vi "Niveau.vi"(8 "error in (no error)":errorcluster, 10 "AngleTable":dbl[](array[numeric]), 11 "Axis entrant":dbl[][](array[numeric])) -> (0 "error out":errorcluster, 3 "Axis sortant":dbl[][](array[numeric]))   [LabVIEW 2019]
uses:
  <vilib>/myRIO/Instrument Drivers/Onboard IO/DIO/typedefs/DIO Reference.ctl
  <vilib>/myRIO/Common/Instrument Driver Framework/Utilities/typedefs/myRIO Generic Hardware Reference.ctl
  <vilib>/myRIO/Common/Instrument Driver Framework/Utilities/typedefs/Hardware Version Enum.ctl
  <vilib>/myRIO/Common/Instrument Driver Framework/Utilities/typedefs/myRIO v1.0 Reference.ctl
  <vilib>/myRIO/Common/Instrument Driver Framework/Utilities/typedefs/Generic FPGA Reference.ctl
  <vilib>/myRIO/Common/Instrument Driver Framework/myRIO v1.0/DIO/typedefs/DIO Channels List.ctl
  <vilib>/myRIO/Common/Instrument Driver Framework/myRIO v1.0/DIO/typedefs/DIO Channels Enum.ctl
  <vilib>/userDefined/High Color/nirio_resource_hc.ctl
  <vilib>/myRIO/Common/Instrument Driver Framework/Utilities/vis/Is FPGA Ref Available.vi
  <vilib>/myRIO/Common/Instrument Driver Framework/myRIO v1.0/DIO/vis/myRIO v1.1 Open DIO.vi
  <vilib>/myRIO/Instrument Drivers/Onboard IO/DIO/vis/Write.vi
  <vilib>/myRIO/Common/Instrument Driver Framework/Utilities/vis/Validate Channels.vi
  <vilib>/myRIO/Common/Instrument Driver Framework/myRIO v1.0/DIO/vis/myRIO v1.0 Reserve DIO.vi
  <vilib>/myRIO/Common/Instrument Driver Framework/myRIO v1.0/Resource Manager/vis/myRIO v1.0 Reserve Channel List.vi
  <vilib>/myRIO/Common/Instrument Driver Framework/myRIO v1.0/DIO/vis/myRIO v1.0 Build MUX Configuration DIO.vi
  <vilib>/myRIO/Common/Instrument Driver Framework/myRIO v1.0/Resource Manager/vis/myRIO v1.0 Reserve Channel.vi
  <vilib>/myRIO/Common/Instrument Driver Framework/myRIO v1.0/Resource Manager/vis/myRIO v1.0 Unreserve Channel.vi
  <vilib>/myRIO/Common/Instrument Driver Framework/myRIO v1.0/Resource Manager/vis/myRIO v1.0 Create Configuration List.vi
  <vilib>/myRIO/Common/Instrument Driver Framework/myRIO v1.0/Resource Manager/vis/myRIO v1.0 Build Mutex Name.vi
  <vilib>/Utility/VariantDataType/GetNumericInfo.vi
  <vilib>/Utility/error.llb/Error Cluster From Error Code.vi
  <vilib>/myRIO/Common/Instrument Driver Framework/myRIO v1.0/myRIO v1.1 Open.vi
  <vilib>/myRIO/Common/Instrument Driver Framework/Utilities/vis/IO Manager.vi
  <vilib>/myRIO/Common/Instrument Driver Framework/Utilities/vis/Configuration Manager.vi
  <vilib>/myRIO/Common/Instrument Driver Framework/myRIO v1.0/Resource Manager/vis/myRIO v1.0 Configure IO.vi
  <vilib>/myRIO/Common/Instrument Driver Framework/myRIO v1.0/myRIO v1.0 Close.vi
  <vilib>/myRIO/Common/Instrument Driver Framework/myRIO v1.0/DIO/vis/myRIO v1.0 Write DIO.vi
  <vilib>/myRIO/Express VI/Onboard Devices/LED/LED Express VI.xnode
  <vilib>/myRIO/Instrument Drivers/Onboard IO/DIO/vis/myRIO DIO Open.xnode
  <vilib>/myRIO/Instrument Drivers/Onboard IO/DIO/DIO.lvlib
panel:
  out "DefAngle":dbl
  out "++Angle":dbl
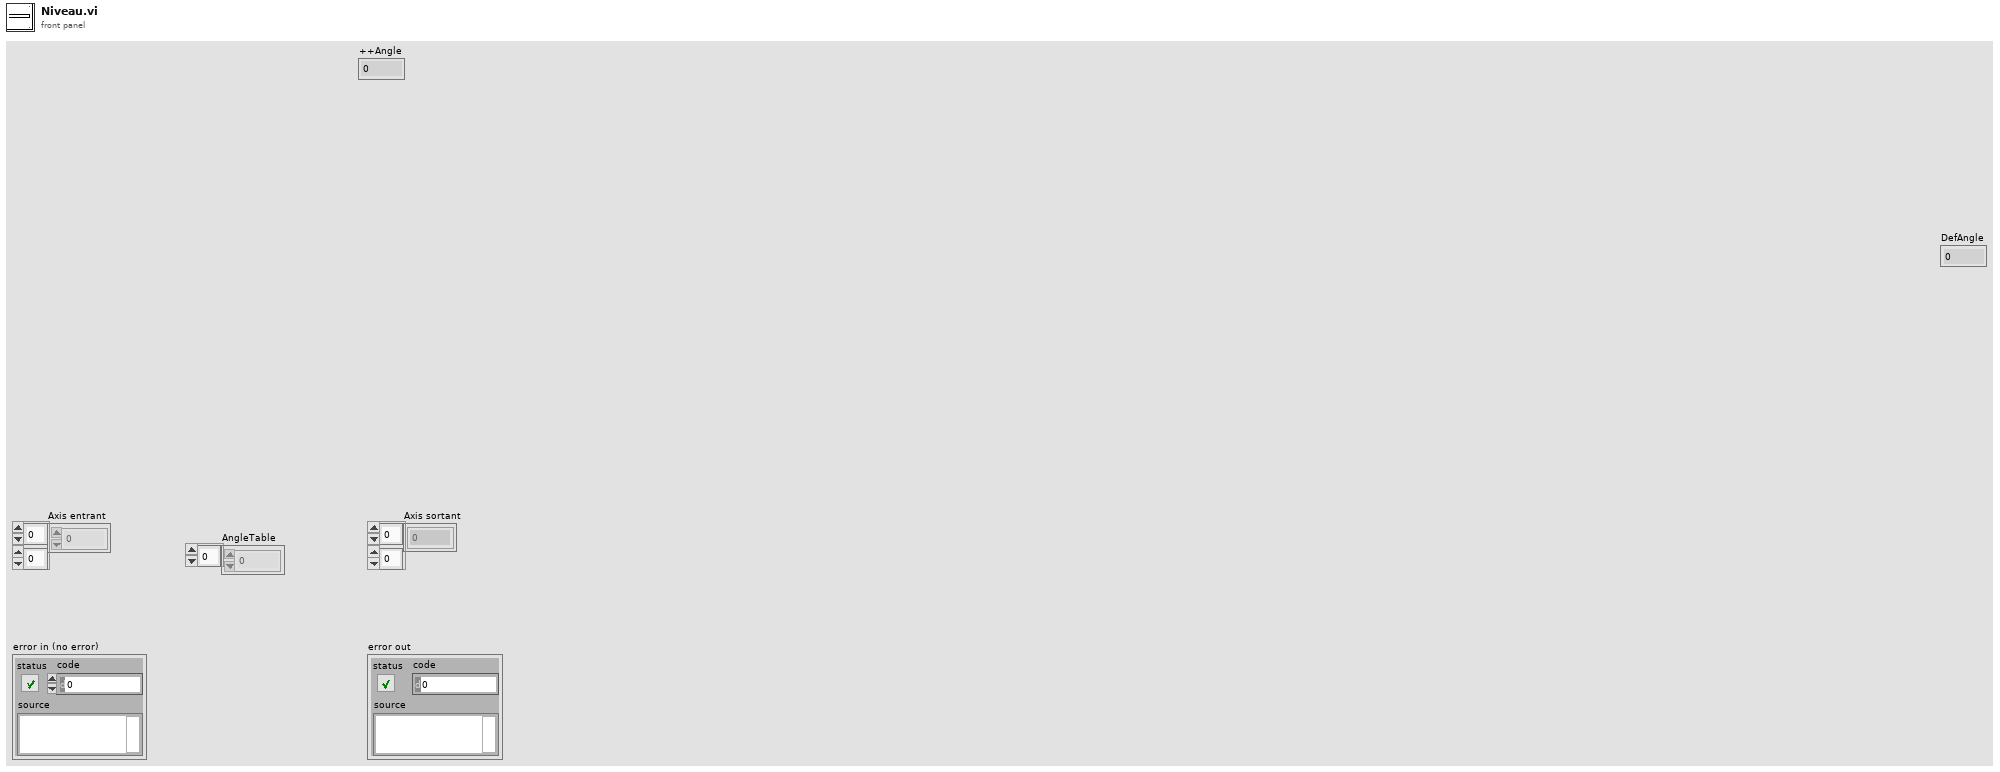
[diagram p1: front panel]
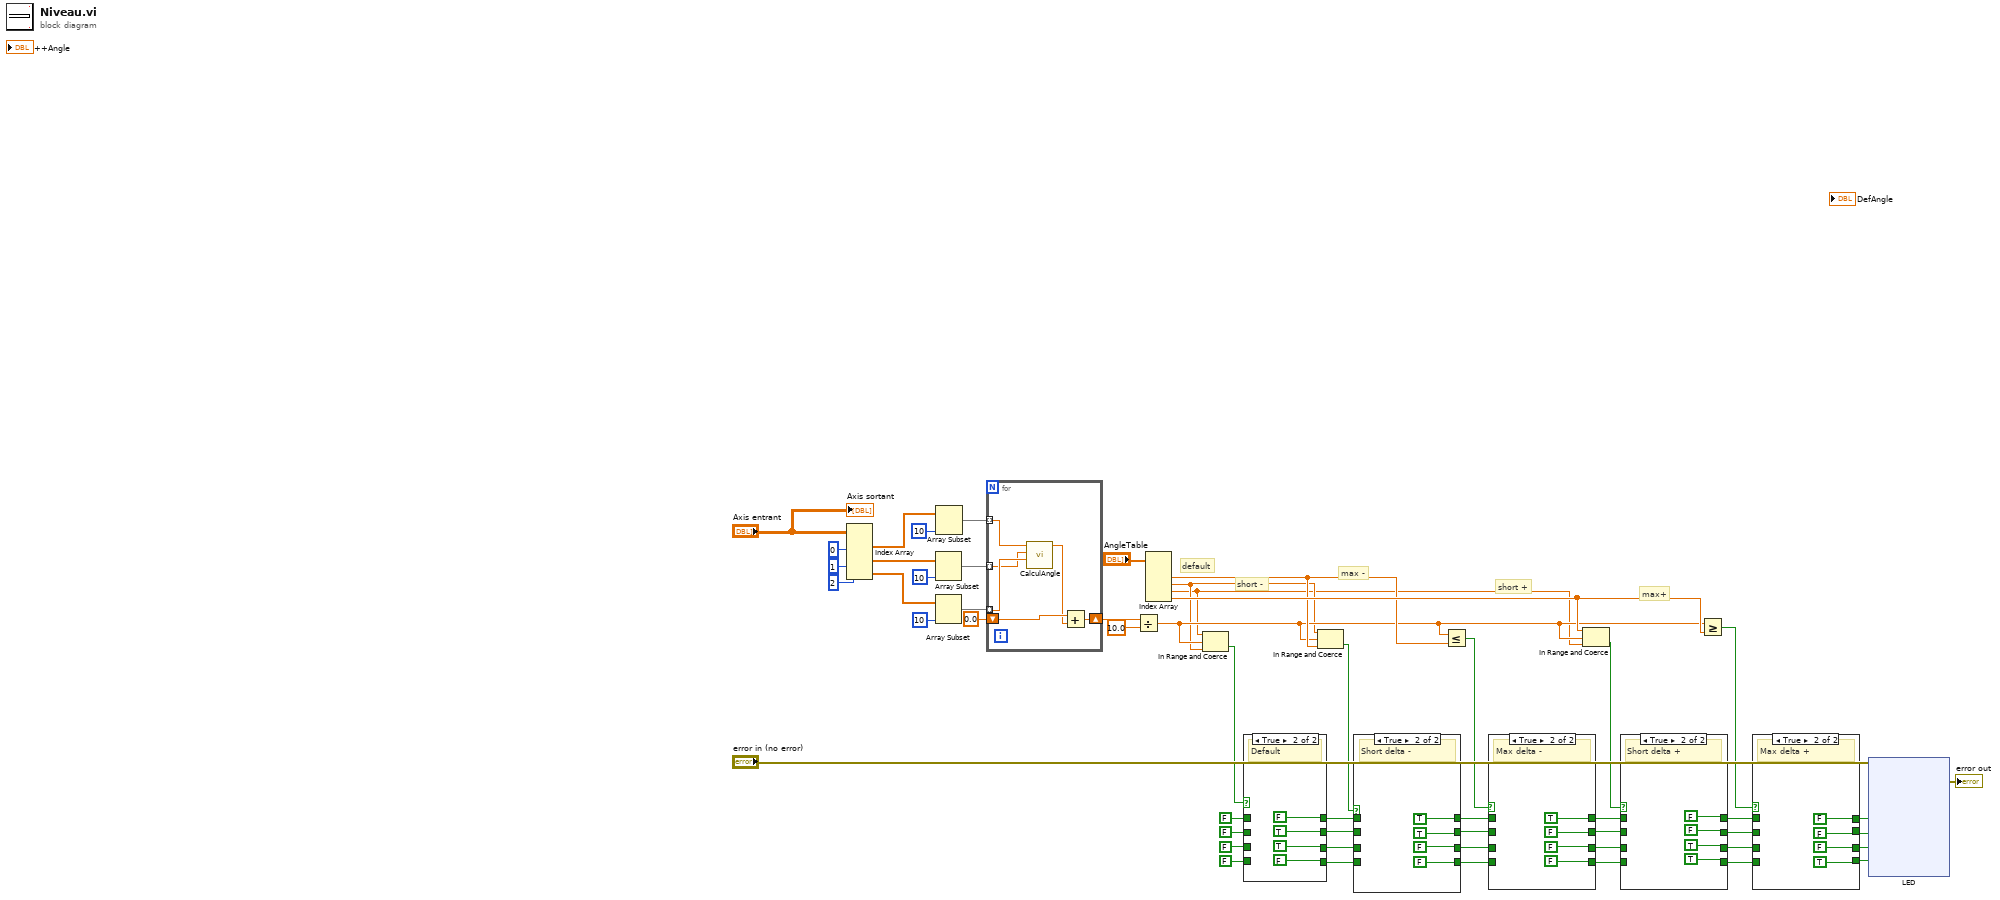
[diagram p0: block diagram]
diagram:
  # "max+"
  # "short +"
  # "short -"
  # "max -"
  # "default"
  n1 = Index Array(array="Axis entrant", index (col) #1=0 ("disabled index (col)"), index (col) #2=1 ("index (col)"), index (col) #3=2 ("index (col)")) -> (element #1=w2:dbl[], element #2=w48:dbl[], element #3=w49:dbl[])  [unwired: 3 in]
  n2 = Array Subset(array=w48, length=10) -> (w51:dbl[])  [unwired: 1 in]
  n3 = Array Subset(array=w49, length=10) -> (w43:dbl[])  [unwired: 1 in]
  n4 = Array Subset(array=w2, length=10) -> (w50:dbl[])  [unwired: 1 in]
  n5 = for {
    tunnel: w43 -> [w56] mode=indexing
    shift-right: [w59] -> w41
    shift-left: 0.0 -> [w58]
    tunnel: w50 -> [w57] mode=indexing
    tunnel: w51 -> [w55] mode=indexing
    n6 = call "CalculAngle.vi"("Zaxis"=w56, "Yaxis"=w55, "Xaxis"=w57) -> ("Numeric"=w54:dbl)  [unwired: 7 in, 1 out]
    n7 = Add(x=w58, y=w54) -> (x+y=w59:dbl)
  }
  n8 = Divide(x=w41, y=10.0) -> (x/y=w6:dbl)
  n9 = Index Array(array="AngleTable") -> (element #2=w7:dbl, element #3=w4:dbl, element #4=w3:dbl, element #5=w8:dbl)  [unwired: 5 in, 1 out]
  n10 = In Range and Coerce(upper limit=w3, x=w6, lower limit=w4) -> (In Range?=w5:bool)  [unwired: 1 out]
  n11 = case shown="True" w5 {
    tunnel: FALSE -> [w63 _]
    tunnel: FALSE -> [w62 _]
    tunnel: FALSE -> [w61 _]
    tunnel: FALSE -> [w60 _]
    tunnel: [w63 FALSE] -> w29
    tunnel: [w62 TRUE] -> w28
    tunnel: [w61 TRUE] -> w27
    tunnel: [w60 FALSE] -> w26
    frame False {
    }
    frame True {
      # "Default"
    }
  }
  n12 = In Range and Coerce(upper limit=w4, x=w6, lower limit=w7) -> (In Range?=w37:bool)  [unwired: 1 out]
  n13 = case shown="True" w37 {
    tunnel: w29 -> [w71 _]
    tunnel: w28 -> [w70 _]
    tunnel: w27 -> [w69 _]
    tunnel: w26 -> [w68 _]
    tunnel: [w71 TRUE] -> w25
    tunnel: [w70 TRUE] -> w20
    tunnel: [w69 FALSE] -> w17
    tunnel: [w68 FALSE] -> w14
    frame False {
    }
    frame True {
      # "Short delta -"
    }
  }
  n14 = Less Or Equal?(x=w6, y=w7) -> (x <= y?=w36:bool)
  n15 = case shown="True" w36 {
    tunnel: w25 -> [w79 _]
    tunnel: [w79 TRUE] -> w24
    tunnel: [w78 FALSE] -> w21
    tunnel: w20 -> [w78 _]
    tunnel: [w77 FALSE] -> w18
    tunnel: w17 -> [w77 _]
    tunnel: [w76 FALSE] -> w15
    tunnel: w14 -> [w76 _]
    frame False {
    }
    frame True {
      # "Max delta -"
    }
  }
  n16 = In Range and Coerce(upper limit=w8, x=w6, lower limit=w3) -> (In Range?=w35:bool)  [unwired: 1 out]
  n17 = case shown="True" w35 {
    tunnel: w24 -> [w87 _]
    tunnel: [w87 FALSE] -> w23
    tunnel: [w86 FALSE] -> w22
    tunnel: w21 -> [w86 _]
    tunnel: [w85 TRUE] -> w19
    tunnel: w18 -> [w85 _]
    tunnel: [w84 TRUE] -> w16
    tunnel: w15 -> [w84 _]
    frame False {
    }
    frame True {
      # "Short delta +"
    }
  }
  n18 = Greater Or Equal?(x=w6, y=w8) -> (x >= y?=w34:bool)
  n19 = case shown="True" w34 {
    tunnel: [w95 FALSE] -> w13
    tunnel: w23 -> [w95 _]
    tunnel: [w94 FALSE] -> w12
    tunnel: w22 -> [w94 _]
    tunnel: [w93 FALSE] -> w11
    tunnel: w19 -> [w93 _]
    tunnel: [w92 TRUE] -> w10
    tunnel: w16 -> [w92 _]
    frame False {
    }
    frame True {
      # "Max delta +"
    }
  }
  n20 = xnode "LED"("LED0"=w13, "LED1"=w12, "LED2"=w11, "LED3"=w10, "error in (no error)"="error in (no error)") -> ("error out"=→"error out":errorcluster)
  "Axis sortant" <- "Axis entrant"
